vi "Drive Train.vi"(0 "C":dbl format="%#_13g", 1 "D":dbl format="%#_13g", 2 "X":dbl format="%#_13g", 3 "Y":dbl format="%#_13g", 4 "gyro":dbl, 6 "Mode Switch":bool, 7 "Positive 1":bool, 9 "Negative 1":bool=TRUE) -> (12 "gyro angle":dbl, 14 "A":dbl, 15 "B":dbl, 16 "R":dbl format="%#_13g")   [LabVIEW 2014]
uses:
  <vilib>/addons/control/pid/pid.llb/PID Advanced (DBL).vi
  <vilib>/addons/control/pid/NI_PID_pid.lvlib
panel:
  in  "dt (s)":dbl=-1.0 format="%.3f"
  in  "derivative time (Td, min)":dbl
  in  "integral time (Ti, min)":dbl
  in  "proportional gain (Kc)":dbl
  in  "alpha":dbl=1.0 step=0.1
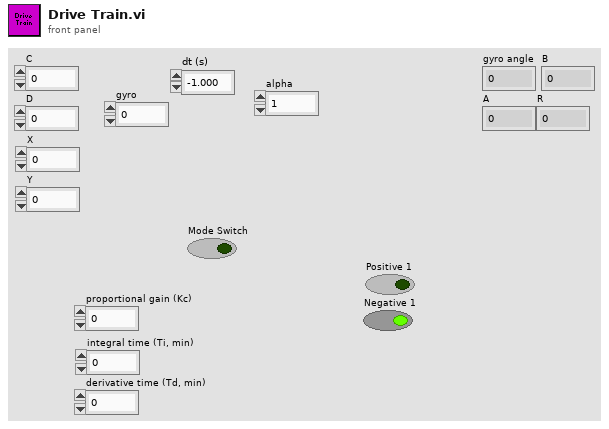
[diagram p1: front panel]
types:
  T1 = cluster{"proportional gain (Kc)":dbl, "integral time (Ti, min)":dbl, "derivative time (Td, min)":dbl}
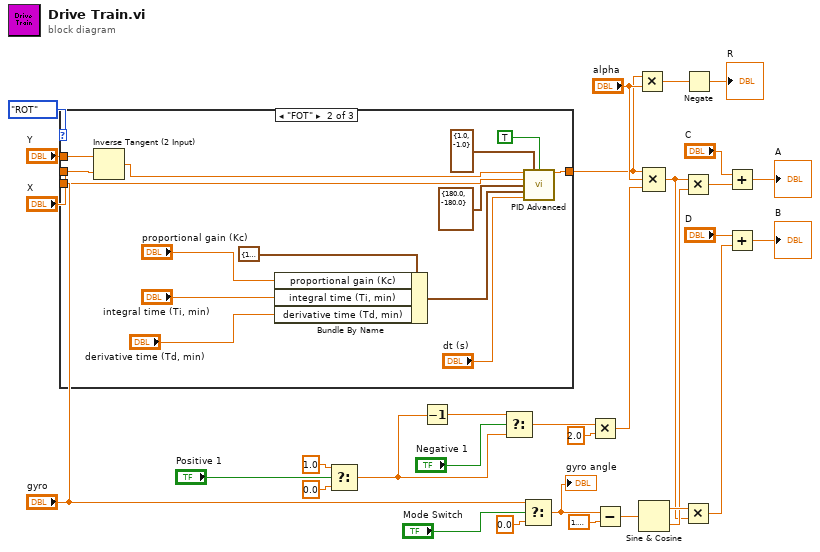
[diagram p0: block diagram]
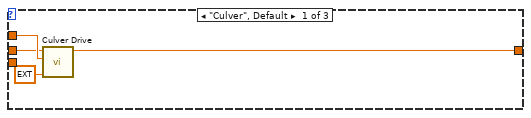
[diagram p2: hidden frame]
diagram:
  n1 = case shown="\"FOT\"" enum16{"ROT", "FOT", "Culver", ""}."ROT" {
    tunnel: "X" -> [w34 w48 w50]
    tunnel: "Y" -> [w35 w49 _]
    tunnel: [w33 w40 w50] -> w2
    tunnel: "gyro" -> [_ w46 _]
    frame "Culver", Default {
      n2 = call "Culver Drive.vi"("Sensitivity"=ext 0.1, "Y"=w35, "X"=w34) -> ("R"=w33:ext)  [unwired: 8 in]
    }
    frame "FOT" {
      n3 = Inverse Tangent (2 Input)(1:w48, 2:w49) -> (0:w47:dbl)
      n4 = Bundle By Name(cluster=T1 {"proportional gain (Kc)"=1.0, "integral time (Ti, min)"=0.01, "derivative time (Td, min)"=0.0} ("PID gains"), "proportional gain (Kc)"="proportional gain (Kc)", "integral time (Ti, min)"="integral time (Ti, min)", "derivative time (Td, min)"="derivative time (Td, min)") -> (w44:T1)
      n5 = call-poly <vilib>:"PID Advanced.vi"("setpoint"=w47, "output range"=cluster{"output high":dbl, "output low":dbl} {"output high"=1.0, "output low"=-1.0}, "auto? (T)"=TRUE, "process variable"=w46, "setpoint range"=cluster{"setpoint high":dbl, "setpoint low":dbl} {"setpoint high"=180.0, "setpoint low"=-180.0}, "PID gains"=w44, "dt (s)"="dt (s)") -> ("output"=w40:dbl)  [unwired: 7 in, 1 out]
    }
    frame "ROT" {
    }
  }
  n6 = Select(t=1.0, s="Positive 1", f=0.0) -> (s? t:f=w19:dbl)
  n7 = Decrement(x=w19) -> (x-1=w18:dbl)
  n8 = Select(t=w18, s="Negative 1", f=w19) -> (s? t:f=w10:dbl)
  n9 = Select(t="gyro", s="Mode Switch", f=0.0 ("t")) -> (s? t:f=w24:dbl)
  "gyro angle" <- w24
  n10 = Multiply(x=w10, y=2.0) -> (x*y=w9:dbl)
  n11 = Subtract(x=w24, y=1.5707963267948966) -> (x-y=w17:dbl)
  n12 = Multiply(x=w2, y="alpha") -> (x*y=w7:ext)
  n13 = Sine & Cosine(0:w17) -> (1:w15:dbl, 2:w12:dbl)
  n14 = Compound Arithmetic op=MULTIPLY(w2, "alpha", w9) -> (w11:ext)
  n15 = Multiply(x=w11, y=w12) -> (x*y=w13:ext)
  n16 = Multiply(x=w15, y=w11) -> (x*y=w14:ext)
  n17 = Negate(x=w7) -> (-x=→"R":ext)
  n18 = Add(x="C", y=w13) -> (x+y=→"A":ext)
  n19 = Add(x="D", y=w14) -> (x+y=→"B":ext)
